vi "Display-GFV.vi"(7 "Chosen Droplet":i32=7, 8 "error in (no error)":errorcluster, 9 "Color":u32(colorbox)=16776793, 10 "Data in":variant, 11 "?":T3=enum."Get Image Ref for Display") -> (0 "error out":errorcluster, 2 "Image Out":T2(plugin-control), 3 "Data out":variant=variant(cluster{"Image Ref":refnum<image>} {"Image Ref"="Display"}))   [LabVIEW 2015]
doc: "Use this template to build a VI to use as a subVI."
uses:
  DisplayGFVEnum.ctl
  DbEnum.ctl
  DropletDB.ctl
  ConfEnum.ctl
  DisplayDB.ctl
  <vilib>/vision/Image Controls.llb/IMAQ Image.ctl
  <resource>/objmgr/IMAQImage.rc
panel:
  in  "Font, Size & Style":T1={"Desired Font (Application)"=enum."User-specified Font", "[User-specified Font]"={"Font Name"="", "Size"=40, "Strikeout?"=FALSE, "Italic?"=FALSE, "Underline?"=FALSE, "Outline?"=FALSE, "Shadow?"=FALSE, "Bold?"=TRUE, "Rotation Angle"=0.0}, "Horizontal Alignment"=0, "Vertical Alignment"=0} {"Vertical Alignment" items=["Bottom", "Top", "Baseline"]; "Horizontal Alignment" items=["Left", "Center", "Right"]; "[User-specified Font]"."Rotation Angle" format="%.2f"}
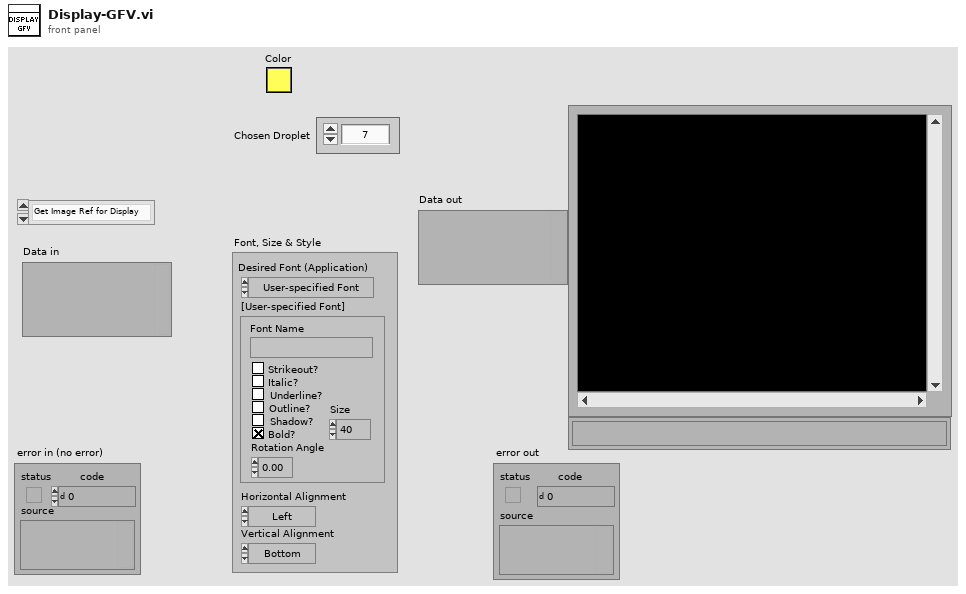
[diagram p1: front panel]
types:
  T1 = cluster{"Desired Font (Application)":enum16{"User-specified Font", "Application Font", "System Font", "Dialog Font"}, "[User-specified Font]":cluster{"Font Name":string, "Size":i16, "Strikeout?":bool, "Italic?":bool, "Underline?":bool, "Outline?":bool, "Shadow?":bool, "Bold?":bool, "Rotation Angle":dbl}, "Horizontal Alignment":i16, "Vertical Alignment":i16}
  T2 = typedef "IMAQ Image.ctl" = refnum<image>
  T3 = typedef "DisplayGFVEnum.ctl" = enum16{"Update Display", "Get Image Ref for Analysis", "Insert Image Ref For Analysis", "Insert Image Ref For Display", "Init Display", "Stop Display", "Get Image Ref for Display"}
  T4 = typedef "ConfEnum.ctl" = enum16{"Insert Threshold Freeze Score", "Insert TolXStd", "ReplacePath", "Init", "GetConfDB", "GetTemperatureAtIndex", "WriteConfDB", "InsertMagnification", "Configure DB"}
  T5 = typedef "DropletDB.ctl" = cluster{"ImageFreezeIndex":i32, "DropIndex":i32, "Position":cluster{"x":sgl, "y":sgl}, "Bounding Box":cluster{"x":sgl, "y":sgl}[], "Score":sgl, "GreyLevelInBoundingBox":dbl[], "GLDifference":dbl[], "Baseline level":dbl, "Peak":cluster{"Value":dbl, "Index":u32}, "Peak Onset":cluster{"Value":dbl, "Index":u32}, "FreezeFileName":string, "FreezeAbsTime":timestamp, "FreezeTemperature":dbl, "ImageIndexArray":u32[], "Freeze Point Found":bool, "Baseline std":dbl, "FreezedImageArray":cluster{"Image":u8[][]}[], "Include Droplet":bool, "Remark":string, "Freeze Rel Time":u32[], "Diameter (microns)":dbl}[]
  T6 = typedef "DbEnum.ctl" = enum16{"RemoveOneDroplet", "AddOneDroplet", "Write DropletDB", "Init", "Insert Detection Result Data", "Insert Grey Level Result", "Insert Baseline Results", "AddFreezeImagesAtCertainDroplet", "UpdateIncludeDroplet", "Insert Freeze Analysis Results", "GetDropDB", "GetNoFreezedDroplets", "GetGreyLevelAndDiff", "GetGreyLevelatIndexTime", "GetDropletsBoundingBox", "GetDropletsDiameter"}
  T7 = typedef "DisplayDB.ctl" = cluster{"Image Ref":T2}
  T8 = cluster{"Array[0]":i32, "Array[1]":i32, "Array[2]":i32, "Array[3]":i32}
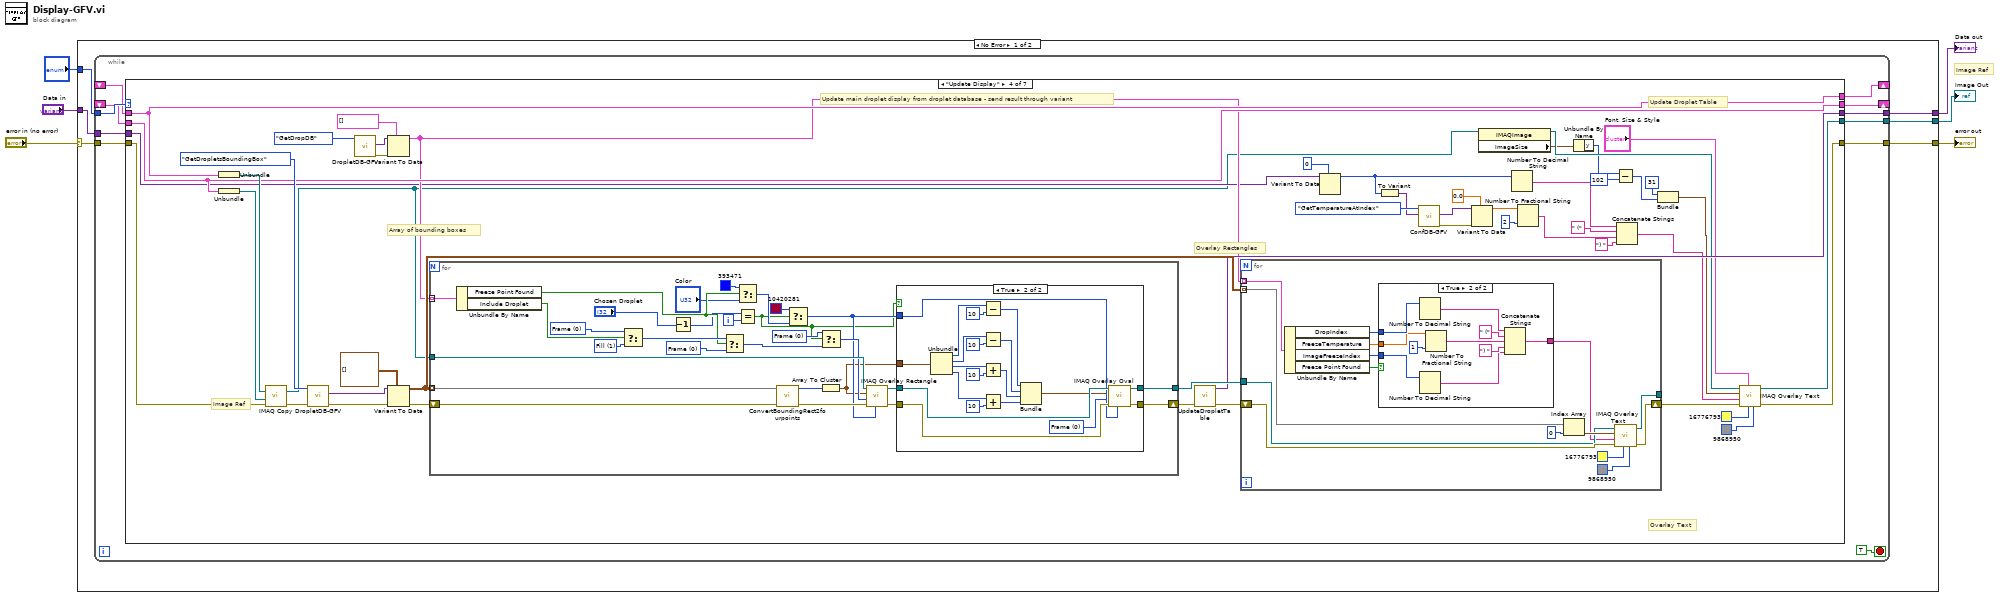
[diagram p0: block diagram]
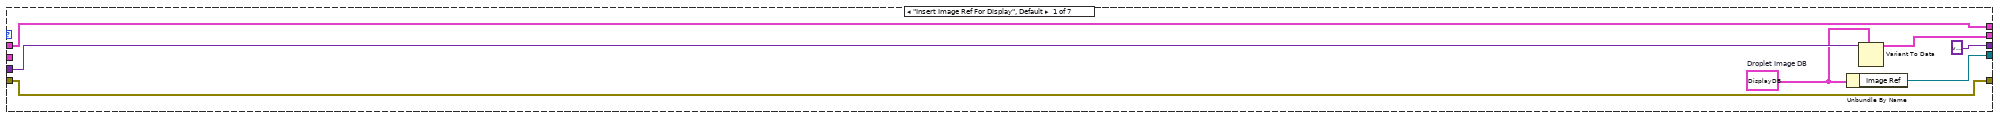
[diagram p2: hidden frame]
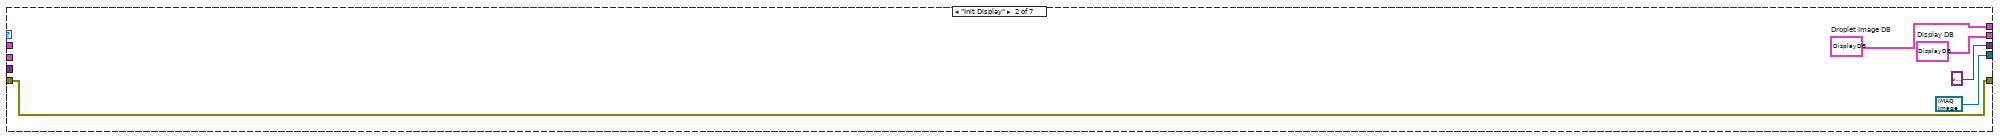
[diagram p3: hidden frame]
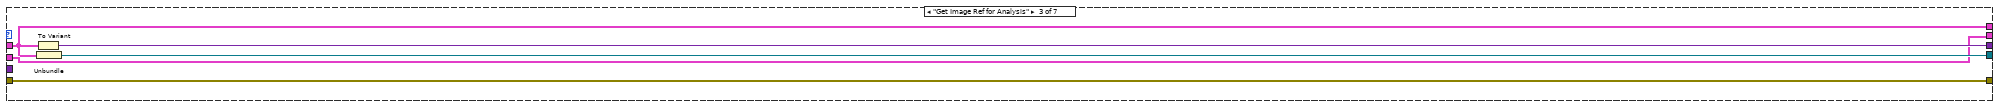
[diagram p4: hidden frame]
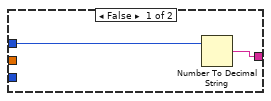
[diagram p5: hidden frame]
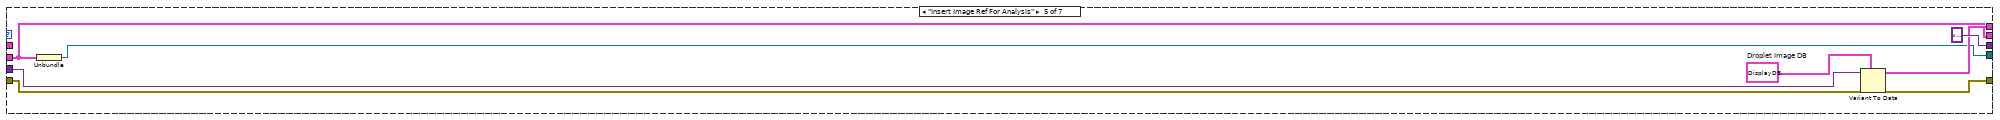
[diagram p7: hidden frame]
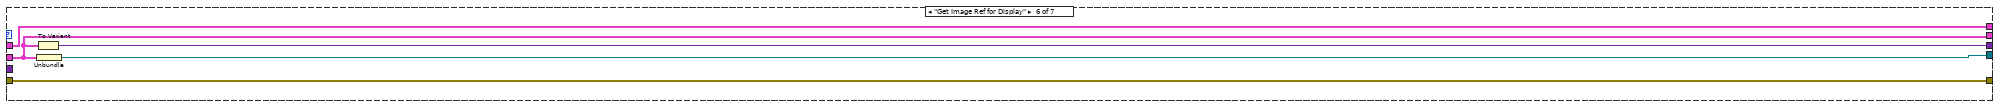
[diagram p8: hidden frame]
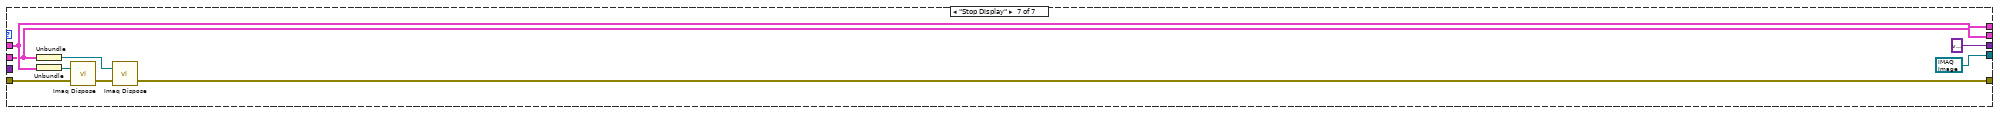
[diagram p9: hidden frame]
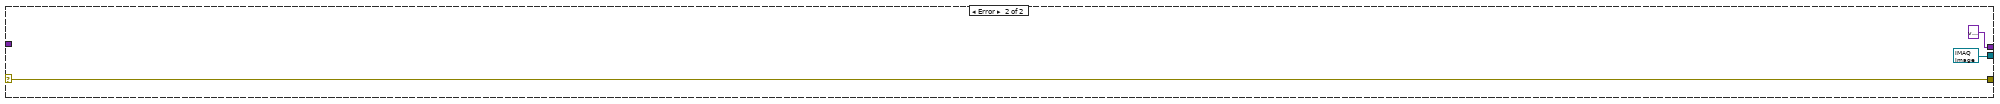
[diagram p10: hidden frame]
diagram:
  # "Image Ref"
  n1 = case shown="No Error" "error in (no error)" {
    selector: "error in (no error)" -> [w9 w193]
    tunnel: [w8 w193] -> w5
    tunnel: "?" -> [w12 _]
    tunnel: "Data in" -> [w11 _]
    tunnel: [w10 variant ("Variant")] -> w2
    tunnel: [w7 T2 refnum ("Image Out")] -> w1
    frame No Error {
      n2 = while {
        tunnel: w12 -> [w22]
        shift-right: [w21] -> _
        shift-left: _ -> [w20]
        tunnel: w11 -> [w19]
        tunnel: [w18] -> w10
        tunnel: w9 -> [w17]
        tunnel: [w16] -> w8
        tunnel: [w15] -> w7
        shift-right: [w14] -> _
        shift-left: _ -> [w13]
        stop <- TRUE stop-if-true
        n3 = case shown="\"Update Display\"" w22 {
          tunnel: [w27 w35 w36 w90 w172 w180 w183] -> w21
          tunnel: w20 -> [w27 _ w36 w90 _ w180 w183]
          tunnel: w19 -> [w30 _ _ w51 w176 _ _]
          tunnel: [variant ("Variant") variant ("Variant") w40 w77 variant ("Variant") w178 variant ("Variant")] -> w18
          tunnel: w17 -> [w28 w33 w39 w80 w174 w179 w188]
          tunnel: [w28 w33 w39 w68 w173 w179 w186] -> w16
          tunnel: [w24 T2 refnum ("Image Out") w38 w67 w171 w181 T2 refnum ("Image Ref")] -> w15
          tunnel: [w29 w31 w37 w82 w170 w177 w182] -> w14
          tunnel: w13 -> [_ _ w37 w82 w170 w177 w182]
          frame "Insert Image Ref For Display", Default {
            w25 = T7 {"Image Ref"=refnum}  # Droplet Image DB
            n4 = Unbundle By Name(w25) -> ("Image Ref"=w24:T2)
            n5 = Variant To Data(type=w25, Variant=w30) -> (data=w29:T7)  [unwired: 1 in, 1 out]
          }
          frame "Init Display" {
            w31 = T7 {"Image Ref"=refnum}  # Display DB
            w35 = T7 {"Image Ref"=refnum}  # Droplet Image DB
          }
          frame "Get Image Ref for Analysis" {
            n6 = To Variant(anything=w36) -> (Variant=w40:variant)
            n7 = Unbundle(w36) -> ("Image Ref"=w38:T2)
          }
          frame "Update Display" {
            # "Update Droplet Table"
            # "Overlay Text"
            # "Overlay Rectangles"
            # "Update main droplet display from droplet database - send result through variant"
            # "Array of bounding boxes"
            # "Image Ref"
            n8 = Unbundle(w90) -> ("Image Ref"=w83:T2)
            n9 = Unbundle(w82) -> ("Image Ref"=w81:T2)
            n10 = call "IMAQ Copy"("error in (no error)"=w80, "Image Dst"=w81, "Image Src"=w83) -> ("error out"=w79:errorcluster, "Image Dst Out"=w48:T2)  [unwired: 3 in]
            n11 = call "DropletDB-GFV.vi"("error in (no error)"=w79, "Command In"=DbEnum."GetDropletsBoundingBox") -> ("error out"=w88:errorcluster, "Data out"=w89:variant)  [unwired: 8 in]
            n12 = call "DropletDB-GFV.vi"("Command In"=DbEnum."GetDropDB") -> ("error out"=w72:errorcluster, "Data out"=w71:variant)  [unwired: 9 in]
            n13 = Variant To Data(error in=w72, type=T5 [] ("DropletArray"), Variant=w71) -> (data=w70:T5)  [unwired: 1 out]
            n14 = Variant To Data(error in=w88, type=cluster{"x":sgl, "y":sgl}[][] [] ("Bounding Box"), Variant=w89) -> (data=w84:cluster{"x":sgl, "y":sgl}[][], error out=w85:errorcluster)
            n15 = for {
              tunnel: w84 -> [w146] mode=indexing
              shift-right: [w121] -> w76
              shift-left: w85 -> [w145]
              tunnel: w48 -> [w144]
              tunnel: [w123] -> w78
              tunnel: w70 -> [w141] mode=indexing
              i -> [w132]
              w126 = u32 0 items=["Frame", "Fill", "Highlight"] ("Drawing Mode (Frame)")
              w134 = u32 0 items=["Frame", "Fill", "Highlight"] ("Drawing Mode (Frame)")
              w137 = u32 0 items=["Frame", "Fill", "Highlight"] ("Drawing Mode (Frame)")
              w138 = u32 1 items=["Frame", "Fill", "Highlight"] ("Drawing Mode (Frame)")
              n16 = Unbundle By Name(w141) -> ("Freeze Point Found"=w135:bool, "Include Droplet"=w139:bool)
              n17 = Select(t=w137, s=w139, f=w138) -> (s? t:f=w136:u32)
              n18 = Decrement(x="Chosen Droplet") -> (x-1=w130:i32)
              n19 = Select(t=w136, s=w135, f=w134) -> (s? t:f=w127:u32)
              n20 = Select(t=u32 393471 ("Color"), s=w135, f="Color") -> (s? t:f=w129:u32)
              n21 = Equal?(x=w130, y=w132) -> (x = y?=w118:bool)
              n22 = call "ConvertBoundingRect2fourpoints.vi"("Error In"=w145, "Bounding Box"=w146) -> ("Error Out"=w142:errorcluster, "Array"=w143:i32[])  [unwired: 8 in]
              n23 = Select(t=u32 10420281 ("Color"), s=w118, f=w129) -> (s? t:f=w120:u32)
              n24 = Select(t=w126, s=w118, f=w127) -> (s? t:f=w125:u32)
              n25 = Array To Cluster(array=w143) -> (cluster=w119:T8)
              n26 = call "IMAQ Overlay Rectangle"("Color"=w120, "error in (no error)"=w142, "Drawing Mode (Frame)"=w125, "Rectangle"=w119, "Image"=w144) -> ("error out"=w122:errorcluster, "Image Out"=w124:T2)  [unwired: 5 in]
              n27 = case shown="True" w118 {
                tunnel: w124 -> [w148 w168]
                tunnel: [w148 w167] -> w123
                tunnel: w122 -> [w147 w166]
                tunnel: [w147 w165] -> w121
                tunnel: w120 -> [_ w164]
                tunnel: w119 -> [_ w163]
                frame False {
                }
                frame True {
                  w149 = u32 0 items=["Frame", "Fill"] ("Drawing Mode (Frame)")
                  n28 = Unbundle(w163) -> ("Array[0]"=w162:i32, "Array[1]"=w159:i32, "Array[2]"=w155:i32, "Array[3]"=w152:i32)
                  n29 = Subtract(x=w162, y=10) -> (x-y=w158:i32)
                  n30 = Subtract(x=w159, y=10) -> (x-y=w157:i32)
                  n31 = Add(x=w155, y=10) -> (x+y=w154:i32)
                  n32 = Add(x=w152, y=10) -> (x+y=w151:i32)
                  n33 = Bundle(w158, w157, w154, w151) -> (w150:cluster{i32, i32, i32, i32})  [unwired: 1 in]
                  n34 = call "IMAQ Overlay Oval"("Color"=w164, "error in (no error)"=w166, "Drawing Mode (Frame)"=w149, "Bounding Rectangle"=w150, "Image"=w168) -> ("error out"=w165:errorcluster, "Image Out"=w167:T2)  [unwired: 5 in]
                }
              }
            }
            n35 = call "UpdateDropletTable.vi"("error in (no error)"=w76) -> ("error out"=w75:errorcluster, "DropletTabeVariant"=w77:variant)  [unwired: 9 in]
            n36 = for {
              tunnel: w84 -> [w103] mode=indexing
              shift-right: [w105] -> w69
              shift-left: w75 -> [w99]
              tunnel: [w104] -> _
              tunnel: w70 -> [w100] mode=indexing
              tunnel: w78 -> [w98]
              n37 = Unbundle By Name(w100) -> ("DropIndex"=w97:i32, "FreezeTemperature"=w96:dbl, "ImageFreezeIndex"=w94:i32, "Freeze Point Found"=w95:bool)
              n38 = case shown="True" w95 {
                tunnel: w97 -> [w107 w117]
                tunnel: w96 -> [_ w114]
                tunnel: w94 -> [_ w112]
                tunnel: [w106 w109] -> w93
                frame False {
                  n39 = Number To Decimal String(number=w107) -> (decimal integer string=w106:string)  [unwired: 1 in]
                }
                frame True {
                  n40 = Number To Decimal String(number=w117) -> (decimal integer string=w116:string)  [unwired: 1 in]
                  n41 = Number To Decimal String(number=w112) -> (decimal integer string=w110:string)  [unwired: 1 in]
                  n42 = Number To Fractional String(number=w114, precision (6)=i16 1) -> (F-format string=w113:string)  [unwired: 2 in]
                  n43 = Concatenate Strings(w116, " (" ("string"), w113, ") " ("string"), w110) -> (w109:string)
                }
              }
              n44 = Index Array(array=w103, index=0) -> (element=w101:cluster{"x":sgl, "y":sgl})
              n45 = call "IMAQ Overlay Text"("BG Color (Transparent)"=u32 9868950, "Text Color (black)"=u32 16776793 ("Color"), "error in (no error)"=w99, "String"=w93, "Origin"=w101, "Image"=w98) -> ("error out"=w105:errorcluster, "Image Out"=w104:T2)  [unwired: 4 in]
            }
            n46 = Variant To Data(type=0, Variant=w51) -> (data=w49:i32)  [unwired: 1 in, 1 out]
            n47 = To Variant(anything=w49) -> (Variant=w62:variant)
            n48 = call "ConfDB-GFV.vi"("Data in"=w62, "Command In"=ConfEnum."GetTemperatureAtIndex") -> ("error out"=w60:errorcluster, "Data out"=w61:variant)  [unwired: 8 in]
            n49 = Variant To Data(error in=w60, type=0.0, Variant=w61) -> (data=w57:dbl)  [unwired: 1 out]
            n50 = property class="IMAQImage"(reference=w48) -> (reference out=w47:T2, "ImageSize"=w46:cluster{"x":i32, "y":i32})  [unwired: 1 in, 1 out]
            n51 = Number To Decimal String(number=w49) -> (decimal integer string=w54:string)  [unwired: 1 in]
            n52 = Number To Fractional String(number=w57, precision (6)=i16 2) -> (F-format string=w53:string)  [unwired: 2 in]
            n53 = Unbundle By Name(w46) -> ("y"=w45:i32)
            n54 = Subtract(x=w45, y=102) -> (x-y=w43:i32)
            n55 = Concatenate Strings(w54, " (" ("string"), w53, ") " ("string")) -> (w52:string)
            n56 = Bundle("X"=31, w43) -> (w41:cluster{"X":i32, i32})  [unwired: 1 in]
            n57 = call "IMAQ Overlay Text"("BG Color (Transparent)"=u32 9868950, "Text Color (black)"=u32 16776793 ("Color"), "Font, Size & Style"="Font, Size & Style", "error in (no error)"=w69, "String"=w52, "Origin"=w41, "Image"=w47) -> ("error out"=w68:errorcluster, "Image Out"=w67:T2)  [unwired: 3 in]
          }
          frame "Insert Image Ref For Analysis" {
            w169 = T7 {"Image Ref"=refnum}  # Droplet Image DB
            n58 = Unbundle(w170) -> ("Image Ref"=w171:T2)
            n59 = Variant To Data(error in=w174, type=w169, Variant=w176) -> (data=w172:T7, error out=w173:errorcluster)
          }
          frame "Get Image Ref for Display" {
            n60 = To Variant(anything=w177) -> (Variant=w178:variant)
            n61 = Unbundle(w177) -> ("Image Ref"=w181:T2)
          }
          frame "Stop Display" {
            n62 = Unbundle(w182) -> ("Image Ref"=w189:T2)
            n63 = Unbundle(w183) -> ("Image Ref"=w190:T2)
            n64 = call "Imaq Dispose"("Image"=w190, "error in (no error)"=w188) -> ("error out"=w187:errorcluster)  [unwired: 4 in]
            n65 = call "Imaq Dispose"("Image"=w189, "error in (no error)"=w187) -> ("error out"=w186:errorcluster)  [unwired: 4 in]
          }
        }
      }
    }
    frame Error {
    }
  }
  "error out" <- w5
  "Data out" <- w2
  "Image Out" <- w1
